vi "Periodic Tasks.vi"(8 "error in":errorcluster) -> ()   [LabVIEW 2015]
doc: "This VI runs in parallel to other tasks. It can contain as many user-defined periodic loops as you need. These can carry out PID or other sorts of timed response."
uses:
  <vilib>/Rock Robotics/WPI/Utilities/WPI_GetSetVariantRefNum.vi
  <vilib>/Rock Robotics/WPI/Ultrasonic/WPI_SonarMB1010DigitalRefNum Registry Get.vi
  <vilib>/Rock Robotics/WPI/Ultrasonic/WPI_SonarMB1010DigitalGetRange.vi
  <vilib>/Rock Robotics/Network Tables/NT Write Number.vi
  Robot Global Data.vi
panel:
  in  "stop 2":bool
  out "X Acceleration 2":dbl
  out "Y Acceleration 2":dbl
  out "Z Acceleration 2":dbl
  out "error out 2":errorcluster
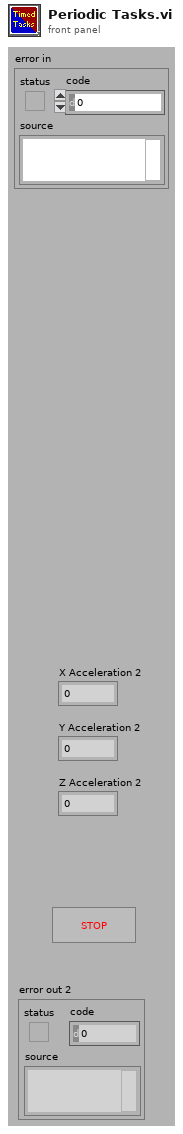
[diagram p1: front panel]
types:
  T1 = typedef "WPI_JoystickDevRef.ctl" = cluster{"Device":T2}
  T2 = typedef "WPI_JoystickDeviceEnum.ctl" = enum16{"USB 0", "USB 1", "USB 2", "USB 3", "USB 4", "USB 5"}
  T3 = typedef "WPI_MotorControlDeviceRef.ctl" = cluster{"DeviceStatus":errorcluster, "Type":T4, "PWM":cluster{"PWM Channel":T5, "DeadBand":T6}, "CAN":cluster{"Device Number":u8, "Control Mode":T7, "Semaphore":T8, "Max Vout":dbl, "TalonSRX Control Mode":T9}, "Invert":bool}
  T4 = typedef "WPI_MotorControlType.ctl" = enum16{"PWM", "CAN", "CANTalonSRX"}
  T5 = typedef "FPGA_DIOPWMChannel.ctl" = enum8{"PWM 0", "PWM 1", "PWM 2", "PWM 3", "PWM 4", "PWM 5", "PWM 6", "PWM 7", "PWM 8", "PWM 9", "PWM MXP 0", "PWM MXP 1", "PWM MXP 2", "PWM MXP 3", "PWM MXP 4", "PWM MXP 5", "PWM MXP 6", "PWM MXP 7", "PWM MXP 8", "PWM MXP 9", "Invalid"}
  T6 = typedef "WPI_PWMDeadband.ctl" = cluster{"Name":string, "maxPositivePwm":i32, "minPositivePwm":i32, "centerPwm":i32, "maxNegativePwm":i32, "minNegativePwm":i32, "angularRange":u16}
  T7 = typedef "WPI_CANJaguar_ControlMode.ctl" = enum8{"Percent VBus", "Current", "Speed", "Position", "Voltage"}
  T8 = typedef "Semaphore RefNum" = refnum<k1>
  T9 = typedef "WPI_CANTalonSRX_APIControlMode.ctl" = enum8{"Percent VBus", "Speed", "Position", "Slave", "Unchanged / Invalid", "Voltage Compensation", "Current", "Motion Profile"}
  T10 = typedef "WPI_ServoDeviceRef.ctl" = cluster{"DeviceStatus":errorcluster, "PWM Channel":T5, "DeadBand":T6}
  T11 = typedef "WPI_AccelerometerDevRef.ctl" = cluster{"DevStatus":errorcluster, "Scaling":T12, "Analog Channels":T13, "I2C Bus":T15, "SPI Bus":T16, "Accel Range":T17, "ADXL Axes":T18, "Handle":i32, "Device Address":u8, "Accel Type":enum16{"Analog", "ADXL345 I2C", "ADXL345 SPI", "Internal", "ADXL362 SPI"}}
  T12 = typedef "WPI_AccelerometerScaling.ctl" = cluster{"Gain (VoltsPerG)":dbl, "Center Voltage":dbl}
  T13 = typedef "WPI_AccelerometerAnalogChannels.ctl" = cluster{"X-Axis":T14, "Y-Axis":T14, "Z-Axis":T14}
  T14 = typedef "FPGA_AIChannel.ctl" = enum8{"AI 0", "AI 1", "AI 2", "AI 3", "AI MXP 0", "AI MXP 1", "AI MXP 2", "AI MXP 3", "Invalid"}
  T15 = typedef "i2c_bus.ctl" = enum16{"I2C On-Board", "I2C MXP", "Invalid"}
  T16 = typedef "spi_bus.ctl" = enum16{"SPI On-Board, CS0", "SPI On-Board, CS1", "SPI On-Board, CS2", "SPI On-Board, CS3", "SPI MXP", "Invalid"}
  T17 = typedef "ADXL345 Range.ctl" = u8
  T18 = typedef "WPI_AccelerometerADXL345 Axes.ctl" = cluster{"X-Axis":bool, "Y-Axis":bool, "Z-Axis":bool}
  T19 = cluster{"JoystickDevRef":T1, "JoystickDevRef":T1, "MotorControlDevRef":T3, "MotorControlDevRef":T3, "MotorControlDevRef":T3, "MotorControlDevRef":T3, "ServoDeviceRef":T10, "MotorControlDevRef":T3, "MotorControlDevRef":T3, "MotorControlDevRef":T3}
  T20 = cluster{"X-Axis":dbl, "Y-Axis":dbl, "Z-Axis":dbl}
  T21 = typedef "WPI_SonarMB1010DigitalDeviceRef.ctl" = cluster{"CounterDevRef":T22, "Scaling factor (s/in)":dbl}
  T22 = typedef "WPI_CounterDevRef.ctl" = cluster{"DevStatus":errorcluster, "CntIndex":T23}
  T23 = typedef "FPGA_CounterCtrSystemIndex.ctl" = enum8{"Ctr 0", "Ctr 1", "Ctr 2", "Ctr 3", "Ctr 4", "Ctr 5", "Ctr 6", "Ctr 7", "Invalid"}
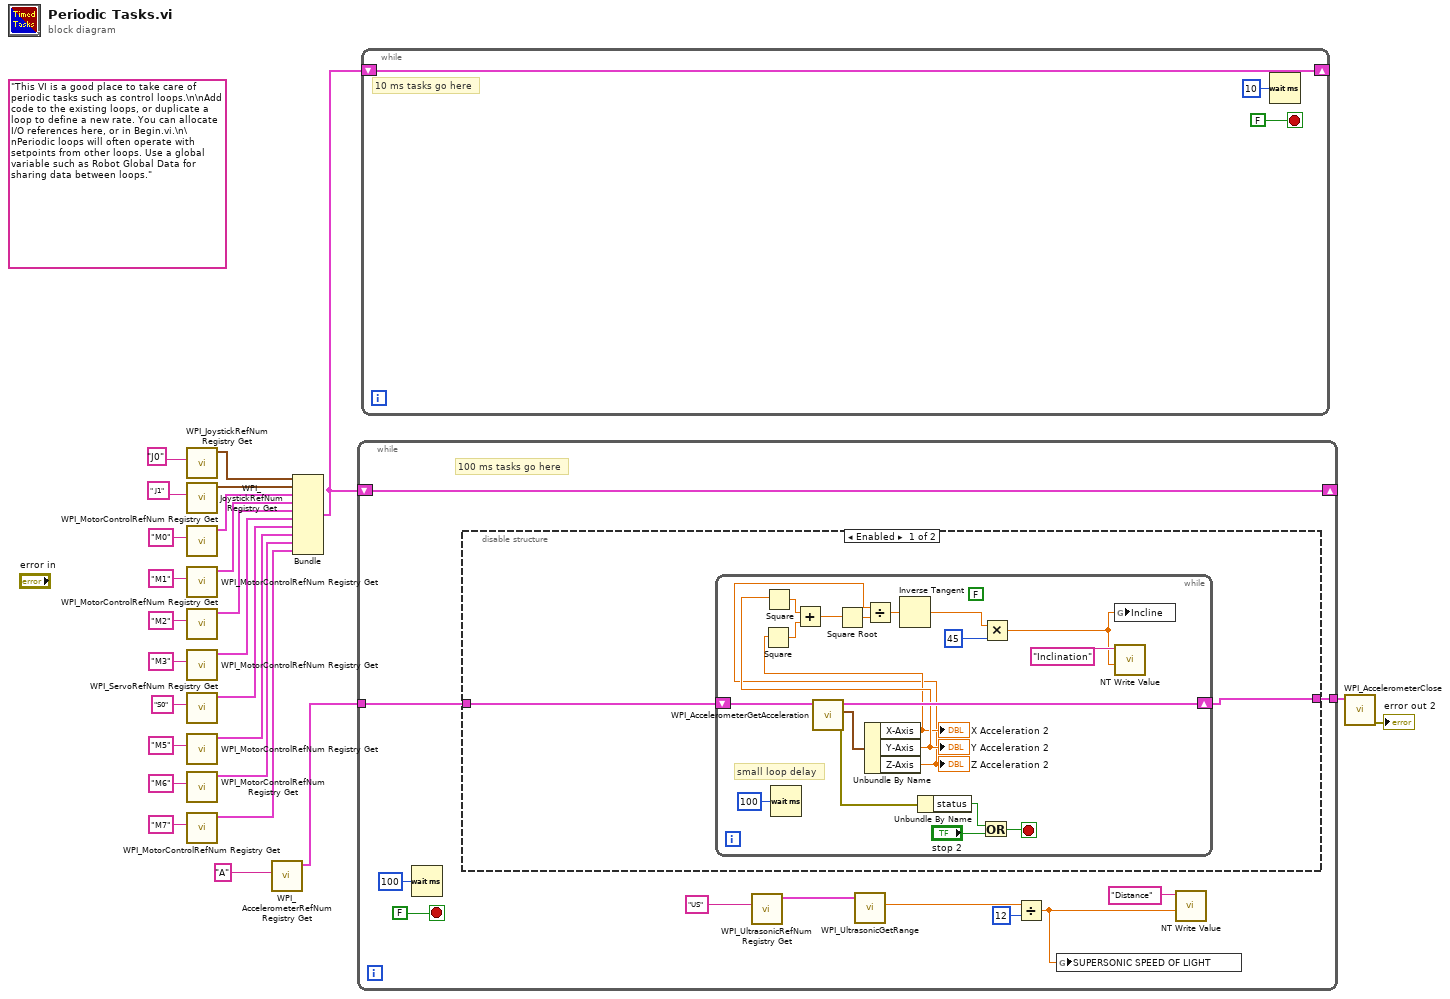
[diagram p0: block diagram]
diagram:
  (unwired) "This VI is a good place to take care of periodic tasks such as control loops.\n\nAdd code to the existing loops, or duplicate a loop to define a new rate. You can allocate I/O references here, or in Begin.vi.\n\nPeriodic loops will often operate with setpoints from other loops. Use a global variable such as Robot Global Data for sharing data between loops."
  n1 = call <vilib>:"WPI_JoystickRefNum Registry Get.vi"("refnum name"="J0") -> ("JoystickDevRef"=w19:T1)  [unwired: 1 in, 9 out]
  n2 = call <vilib>:"WPI_JoystickRefNum Registry Get.vi"("refnum name"=" J1") -> ("JoystickDevRef"=w24:T1)  [unwired: 1 in, 9 out]
  n3 = call <vilib>:"WPI_MotorControlRefNum Registry Get.vi"("refnum name"="M0") -> ("MotorControlDevRef"=w17:T3)  [unwired: 9 in, 1 out]
  n4 = call <vilib>:"WPI_MotorControlRefNum Registry Get.vi"("refnum name"="M1") -> ("MotorControlDevRef"=w21:T3)  [unwired: 9 in, 1 out]
  n5 = call <vilib>:"WPI_MotorControlRefNum Registry Get.vi"("refnum name"="M2") -> ("MotorControlDevRef"=w12:T3)  [unwired: 9 in, 1 out]
  n6 = call <vilib>:"WPI_MotorControlRefNum Registry Get.vi"("refnum name"="M3") -> ("MotorControlDevRef"=w11:T3)  [unwired: 9 in, 1 out]
  n7 = call <vilib>:"WPI_ServoRefNum Registry Get.vi"("refnum name"="S0") -> ("ServoDeviceRef"=w10:T10)  [unwired: 9 in, 1 out]
  n8 = call <vilib>:"WPI_MotorControlRefNum Registry Get.vi"("refnum name"="M5") -> ("MotorControlDevRef"=w9:T3)  [unwired: 9 in, 1 out]
  n9 = call <vilib>:"WPI_MotorControlRefNum Registry Get.vi"("refnum name"="M6") -> ("MotorControlDevRef"=w6:T3)  [unwired: 9 in, 1 out]
  n10 = call <vilib>:"WPI_MotorControlRefNum Registry Get.vi"("refnum name"="M7") -> ("MotorControlDevRef"=w5:T3)  [unwired: 9 in, 1 out]
  n11 = call <vilib>:"WPI_AccelerometerRefNum Registry Get.vi"("refnum name"="A") -> ("AccelerometerDevRef"=w1:T11)  [unwired: 9 in, 1 out]
  n12 = Bundle("JoystickDevRef"=w19, "JoystickDevRef"=w24, "MotorControlDevRef"=w17, "MotorControlDevRef"=w21, "MotorControlDevRef"=w12, "MotorControlDevRef"=w11, "ServoDeviceRef"=w10, "MotorControlDevRef"=w9, "MotorControlDevRef"=w6, "MotorControlDevRef"=w5) -> (w23:T19)  [unwired: 1 out]
  n13 = while {
    shift-right: [w34] -> _
    shift-left: w23 -> [w34]
    tunnel: [w27] -> w3
    tunnel: w1 -> [w26]
    stop <- FALSE stop-if-true
    # "100 ms tasks go here"
    n14 = Wait (ms)(milliseconds to wait=u32 100) -> ()  [unwired: 1 out]
    n15 = disable-structure shown="Enabled" {
      disable-tunnel: [w38 _] -> w27
      disable-tunnel: w26 -> [w37 _]
      frame Enabled {
        (unwired) FALSE
        n16 = while {
          shift-right: [w54] -> w38
          shift-left: w37 -> [w44]
          stop <- w55 stop-if-true
          # "small loop delay"
          n17 = Wait (ms)(milliseconds to wait=u32 100) -> ()  [unwired: 1 out]
          n18 = call <vilib>:"WPI_AccelerometerGetAcceleration.vi"("AccelerometerDevRef"=w44) -> ("error out"=w52:errorcluster, "Accelerations"=w53:T20, "AccelerometerDevRef"=w54:T11)  [unwired: 8 in]
          n19 = Unbundle By Name(w53) -> ("X-Axis"=w43:dbl, "Y-Axis"=w50:dbl, "Z-Axis"=w42:dbl)
          "X Acceleration 2" <- w43
          "Y Acceleration 2" <- w50
          "Z Acceleration 2" <- w42
          n20 = Square(x=w43) -> (x^2=w49:dbl)
          n21 = Square(x=w50) -> (x^2=w48:dbl)
          n22 = Add(x=w48, y=w49) -> (x+y=w47:dbl)
          n23 = Square Root(x=w47) -> (sqrt(x)=w51:dbl)
          n24 = Divide(x=w42, y=w51) -> (x/y=w46:dbl)
          n25 = Inverse Tangent(1:w46) -> (0:w40:dbl)
          n26 = Unbundle By Name(w52) -> ("status"=w58:bool)
          n27 = Or(x=w58, y="stop 2") -> (x .or. y?=w55:bool)
          n28 = Multiply(x=w40, y=45) -> (x*y=w41:dbl)
          n29 = global write "Robot Global Data.vi" "Incline"(w41) -> ()
          n30 = call-poly <vilib>:"NT Write Value.vi"("Numeric"=w41, "Name"="Inclination" ("refnum name")) -> ()  [unwired: 9 in, 1 out]
        }
      }
      frame Disabled {
      }
    }
    n31 = call-poly <vilib>:"WPI_UltrasonicRefNum Registry Get.vi"("refnum name"="US") -> ("SonarMB1010DigitalDevRef"=w33:T21)  [unwired: 9 in, 1 out]
    n32 = call-poly <vilib>:"WPI_UltrasonicGetRange.vi"("SonarMB1010DigitalDevRef"=w33) -> ("Distance"=w30:dbl)  [unwired: 8 in, 2 out]
    n33 = Divide(x=w30, y=12) -> (x/y=w28:dbl)
    n34 = global write "Robot Global Data.vi" "SUPERSONIC SPEED OF LIGHT"(w28) -> ()
    n35 = call-poly <vilib>:"NT Write Value.vi"("Numeric"=w28, "Name"="Distance" ("refnum name")) -> ()  [unwired: 9 in, 1 out]
  }
  n36 = while {
    shift-right: [w59] -> _
    shift-left: w23 -> [w59]
    stop <- FALSE stop-if-true
    # "10 ms tasks go here"
    n37 = Wait (ms)(milliseconds to wait=u32 10) -> ()  [unwired: 1 out]
  }
  n38 = call <vilib>:"WPI_AccelerometerClose.vi"("AccelerometerDevRef"=w3) -> ("error out"=→"error out 2":errorcluster)  [unwired: 10 in]
